vi "caps_lock.vi"() -> ()   [LabVIEW 2023]
panel:
  in  "stop":bool
  in  "Input String":string
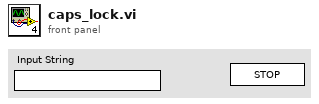
[diagram p1: front panel]
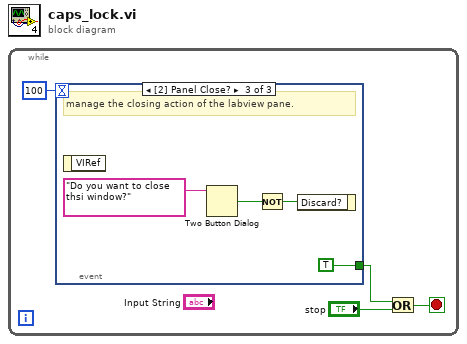
[diagram p0: block diagram]
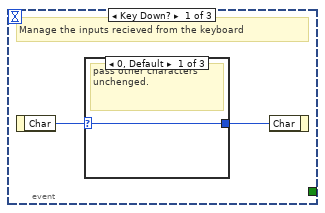
[diagram p2: hidden frame]
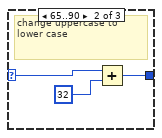
[diagram p3: hidden frame]
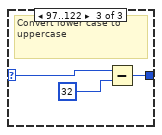
[diagram p4: hidden frame]
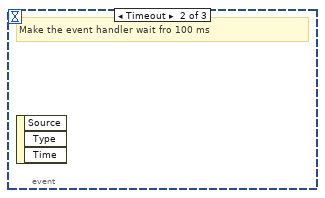
[diagram p5: hidden frame]
diagram:
  n1 = while {
    stop <- w1 stop-if-true
    n2 = event shown="[2] Panel Close?" {
      selector: _ -> [_ _ _]
      dyn-events: _ -> [_ _ _]
      timeout: 100 -> [_ _ _]
      tunnel: [_ _ TRUE] -> w2
      event Key Down? {
        # "Manage the inputs recieved from the keyboard"
        n3 = event-data() -> ("Char"=w6:i16)  [unwired: 1 in]
        n4 = case shown="0, Default" w6 {
          selector: w6 -> [w7 w9 w11]
          tunnel: [w7 w10 w12] -> w5
          frame 0, Default {
            # "pass other characters unchenged."
          }
          frame 65..90 {
            # "change uppercase to lower case"
            n5 = Add(x=w9, y=i16 32) -> (x+y=w10:i16)
          }
          frame 97..122 {
            # "Convert lower case to uppercase"
            n6 = Subtract(x=w11, y=i16 32) -> (x-y=w12:i16)
          }
        }
        n7 = event-data("Char"=w5) -> ()  [unwired: 1 in, 1 out]
      }
      event Timeout {
        # "Make the event handler wait fro 100 ms"
        n8 = event-data() -> ()  [unwired: 1 in, 3 out]
      }
      event Panel Close? {
        # "manage the closing action of the labview pane."
        n9 = event-data() -> ()  [unwired: 1 in, 1 out]
        n10 = Two Button Dialog(message="Do you want to close thsi window?") -> (T button?=w16:bool)  [unwired: 2 in]
        n11 = Not(x=w16) -> (.not. x?=w14:bool)
        n12 = event-data("Discard?"=w14) -> ()  [unwired: 1 in, 1 out]
      }
    }
    n13 = Or(x=w2, y="stop") -> (x .or. y?=w1:bool)
  }
